vi "FitGaussianSpot.vi"() -> ()   [LabVIEW 2014]
uses:
  Globals/AndorImage.vi
panel:
  out "Horizontal Fit Offset":dbl
  out "Horizontal Fit 4*Sigma Width":dbl format="%_2g"
  out "Horizontal Fit Center":dbl format="%_4f"
  out "Horizontal Fit Amplitude":dbl
  out "Vertical Fit 4*Sigma Width":dbl format="%_2g"
  out "Vertical Fit Center":dbl format="%_4g"
  out "Vertical Fit Amplitude":dbl
  out "Vertical Fit Offset":dbl
  out "Horizontal":dbl[][](graph)
  out "Vertical":dbl[][](graph)
  out "Max Value":i32
  in  "Vertical Length":i32=512
  in  "Vertical Start":i32=1
  in  "Horizontal Length":i32=512
  in  "Horizontal Start":i32=1
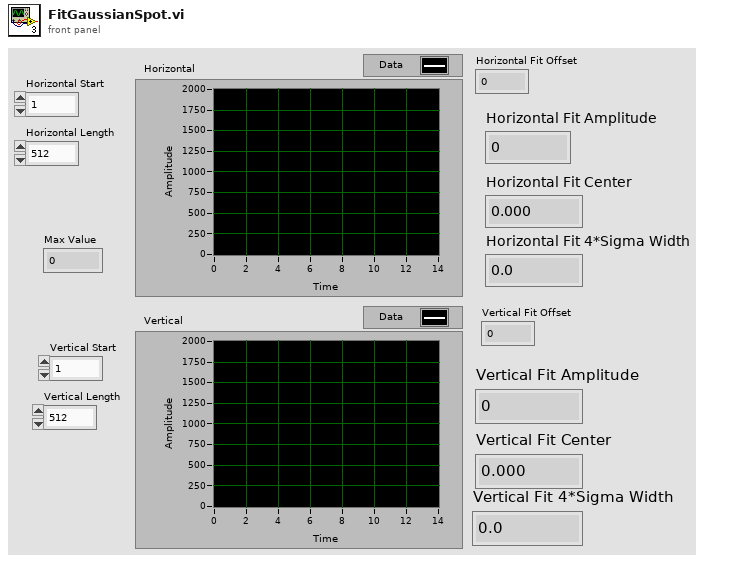
[diagram p1: front panel]
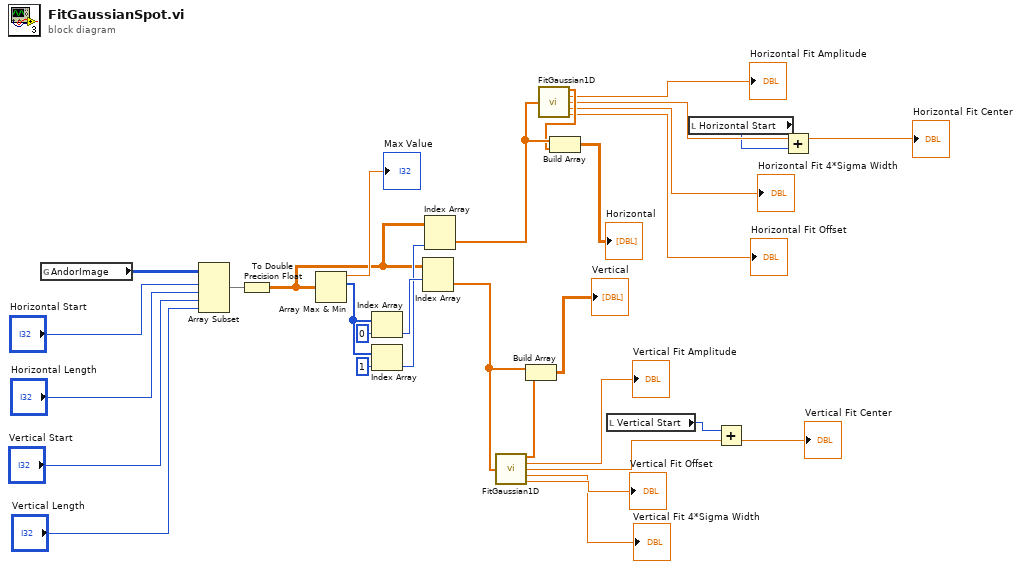
[diagram p0: block diagram]
diagram:
  n1 = global read "AndorImage.vi" "AndorImage"() -> (w31:i32[][])
  n2 = Array Subset(array=w31, index (row)="Horizontal Start", length (row)="Horizontal Length", index (col)="Vertical Start", length (col)="Vertical Length") -> (w20:i32[][])
  n3 = To Double Precision Float(number=w20) -> (double precision float=w1:dbl[][])
  n4 = Array Max & Min(array=w1) -> (max value=→"Max Value":dbl, max index (indices)=w22:i32[])  [unwired: 2 out]
  n5 = Index Array(array=w22, index=0) -> (element=w23:i32)
  n6 = Index Array(array=w22, index=1) -> (element=w21:i32)
  n7 = Index Array(array=w1, index (row)=w23) -> (element=w19:dbl[])  [unwired: 1 in]
  n8 = Index Array(array=w1, index (col)=w21) -> (element=w12:dbl[])  [unwired: 1 in]
  n9 = call "FitGaussian1D.vi"("1D Array to Fit"=w19) -> ("Best Gaussian Fit Array"=w18:dbl[], "Fit Amplitude"=→"Vertical Fit Amplitude":dbl, "Fit Center"=w14:dbl, "Fit 4*Sigma Width"=→"Vertical Fit 4*Sigma Width":dbl, "Fit Offset"=→"Vertical Fit Offset":dbl)  [unwired: 10 in]
  n10 = Build Array(w19, w18) -> (→"Vertical":dbl[][])
  n11 = call "FitGaussian1D.vi"("1D Array to Fit"=w12) -> ("Best Gaussian Fit Array"=w11:dbl[], "Fit Amplitude"=→"Horizontal Fit Amplitude":dbl, "Fit Center"=w8:dbl, "Fit 4*Sigma Width"=→"Horizontal Fit 4*Sigma Width":dbl, "Fit Offset"=→"Horizontal Fit Offset":dbl)  [unwired: 10 in]
  n12 = Build Array(w12, w11) -> (→"Horizontal":dbl[][])
  n13 = local read "Vertical Start"() -> (w4:i32)
  n14 = local read "Horizontal Start"() -> (w2:i32)
  n15 = Add(x=w4, y=w14) -> (x+y=→"Vertical Fit Center":dbl)
  n16 = Add(x=w8, y=w2) -> (x+y=→"Horizontal Fit Center":dbl)
